vi "Get S_n.vi"(10 "n":i32, 11 "Analytical Serial Arm Class in":refnum<class "NI_Robotics_Analytical Serial Arm Class.lvclass">) -> (2 "S_n":dbl, 3 "Analytical Serial Arm Class out":refnum<class "NI_Robotics_Analytical Serial Arm Class.lvclass">)   [LabVIEW 2017, in "NI_Robotics_Analytical Serial Arm Class.lvclass"]
uses:
  <vilib>/robotics/Kinematics/Analytical/Generic/NI_Robotics_Analytical Serial Arm Class.lvclass
  c:/Program Files (x86)/National Instruments/LabVIEW 2017/vi.lib/robotics/Kinematics/Robot/NI_Robotics_Serial Robot Arm.lvclass
  <vilib>/robotics/Kinematics/Link/NI_Robotics_Link.lvclass/NI_Robotics_Link.ctl
  <vilib>/robotics/Kinematics/Analytical/Generic/Accessors/Read S_0.vi
  <vilib>/robotics/Kinematics/Analytical/Generic/Accessors/Read S_n.vi
  <vilib>/robotics/Kinematics/Robot/NI_Robotics_Serial Robot Arm.lvclass
  <vilib>/robotics/Kinematics/Link/NI_Robotics_Link.lvclass
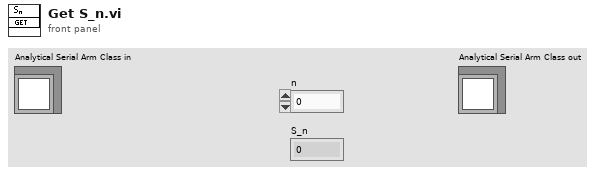
[diagram p1: front panel]
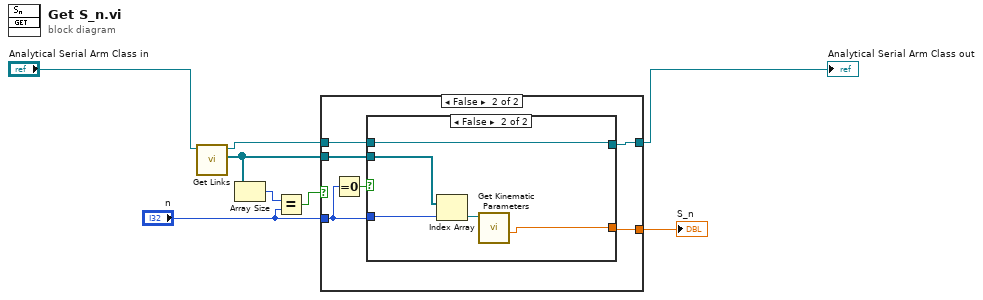
[diagram p0: block diagram]
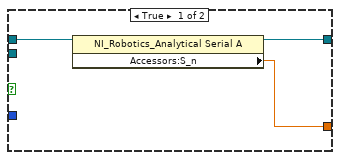
[diagram p2: hidden frame]
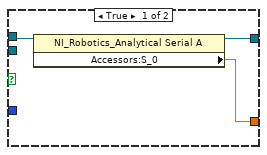
[diagram p3: hidden frame]
diagram:
  n1 = call <vilib>:"Get Links.vi"("serial arm in"="Analytical Serial Arm Class in") -> ("links"=w6:refnum<class "NI_Robotics_Link.lvclass">[], "serial arm out"=w2:refnum<class "NI_Robotics_Analytical Serial Arm Class.lvclass">)  [unwired: 8 in, 1 out]
  n2 = Array Size(array=w6) -> (size(s)=w5:i32)
  n3 = Equal?(x=w5, y="n") -> (x = y?=w3:bool)
  n4 = case shown="False" w3 {
    tunnel: "n" -> [_ w14]
    tunnel: w6 -> [_ w17]
    tunnel: [w10 w16] -> w7
    tunnel: w2 -> [w11 w13]
    tunnel: [w9 w12] -> w1
    frame True {
      n5 = property class="NI_Robotics_Analytical Serial A"(reference=w11) -> (reference out=w9:refnum<class "NI_Robotics_Analytical Serial Arm Class.lvclass">, "Accessors:S_n"=w10:dbl)  [unwired: 1 in, 1 out]
    }
    frame False {
      n6 = Equal To 0?(x=w14) -> (x = 0?=w15:bool)
      n7 = case shown="False" w15 {
        tunnel: w14 -> [_ w25]
        tunnel: w17 -> [_ w23]
        tunnel: [w19 w22] -> w16
        tunnel: w13 -> [w20 w21]
        tunnel: [w18 w21] -> w12
        frame True {
          n8 = property class="NI_Robotics_Analytical Serial A"(reference=w20) -> (reference out=w18:refnum<class "NI_Robotics_Analytical Serial Arm Class.lvclass">, "Accessors:S_0"=w19:dbl)  [unwired: 1 in, 1 out]
        }
        frame False {
          n9 = Index Array(array=w23, index=w25) -> (element=w24:refnum<class "NI_Robotics_Link.lvclass">)
          n10 = call <vilib>:"Get Kinematic Parameters.vi"("NI_Robotics_Link in"=w24) -> ("Offset Distance"=w22:dbl)  [unwired: 6 in, 4 out]
        }
      }
    }
  }
  "Analytical Serial Arm Class out" <- w1
  "S_n" <- w7
